vi "Scale Remote Coordinates to DC Powers.vi"(4 "Deadband (10)":i16=10, 5 "Coord":i8) -> (1 "Power":i16)   [LabVIEW 2012, in "Tetrix.lvlib"]
uses:
  Tetrix.lvlib
  <vilib>/NXT/Dual Mode Library/prims/inRangeAndCoerce/inRangeAndCoerce_int.vi
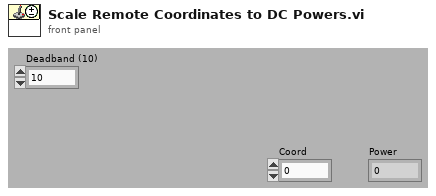
[diagram p1: front panel]
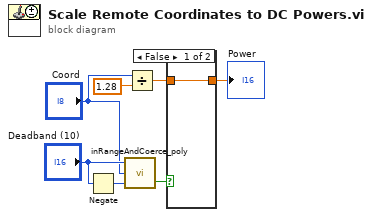
[diagram p0: block diagram]
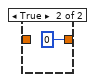
[diagram p2: hidden frame]
diagram:
  n1 = Negate(x="Deadband (10)") -> (-x=w3:i16)
  n2 = call-poly <vilib>:"inRangeAndCoerce_poly.vi"("lower limit"=w3, "x"="Coord", "upper limit"="Deadband (10)") -> ("In Range?"=w6:bool)  [unwired: 1 out]
  n3 = Divide(x="Coord", y=1.28) -> (x/y=w2:dbl)
  n4 = case shown="False" w6 {
    tunnel: w2 -> [w8 _]
    tunnel: [w8 0] -> w5
    frame False {
    }
    frame True {
    }
  }
  "Power" <- w5
